vi "ResMgr-Request StatusEvent.vi"(6 "timeout in ms (5000ms)":i32=5000, 7 "WatchDogQ":refnum<queue>, 8 "Error in":errorcluster caption="Error in (no error)") -> (0 "Error out":errorcluster, 3 "Status Message":refnum<user-event>)   [LabVIEW 2017, in "Communicable State Machine.lvlib"]
uses:
  Communicable State Machine.lvlib
  Typedef/_CSM Status Change Event Data.ctl
  ResMgr-RequestDef.ctl
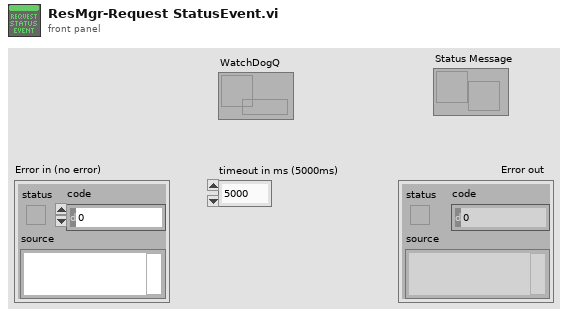
[diagram p1: front panel]
types:
  T1 = typedef "Communicable State Machine.lvlib/ResMgr-RequestDef.ctl" = cluster{"ResType":string, "RespQ":refnum<queue>, "Parameter":string, "WatchDogQ":refnum<queue>}
  T2 = typedef "Communicable State Machine.lvlib/_CSM Status Change Event Data.ctl" = cluster{"ModuleName":string, "Status":string, "Arguments":string}
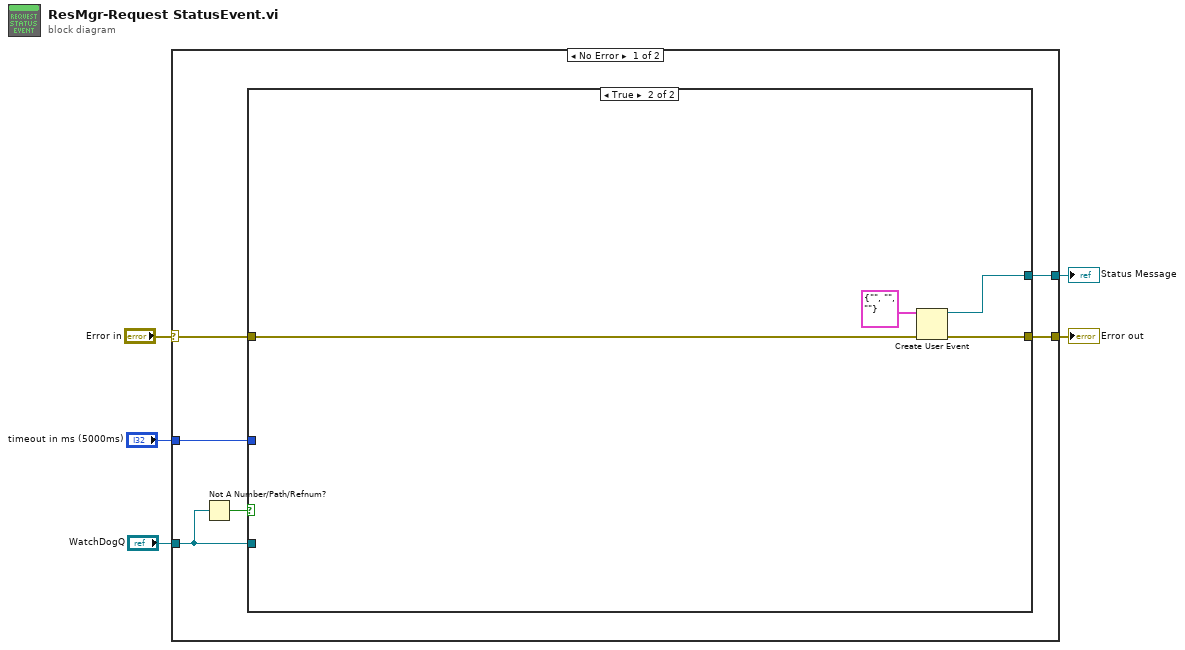
[diagram p0: block diagram]
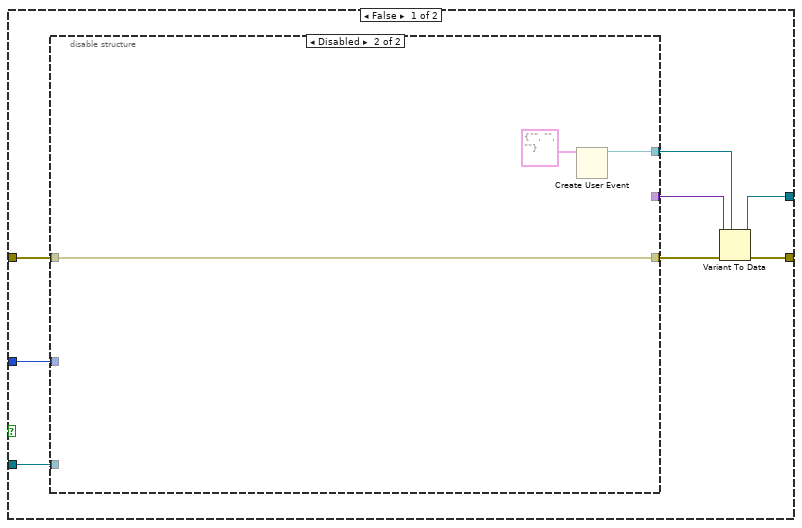
[diagram p2: hidden frame]
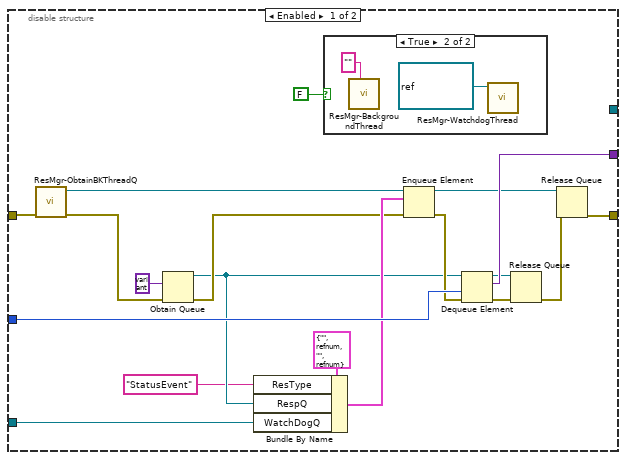
[diagram p3: hidden frame]
diagram:
  n1 = case shown="No Error" "Error in" {
    selector: "Error in" -> [w10 w48]
    tunnel: [w9 w48] -> w5
    tunnel: [w8 _] -> w1
    tunnel: "timeout in ms (5000ms)" -> [w11 _]
    tunnel: "WatchDogQ" -> [w6 _]
    frame No Error {
      n2 = Not A Number/Path/Refnum?(number/path/refnum=w6) -> (NaN/Path/Refnum?=w7:bool)
      n3 = case shown="True" w7 {
        tunnel: w11 -> [w18 _]
        tunnel: w10 -> [w17 w45]
        tunnel: w6 -> [w16 _]
        tunnel: [w15 w46] -> w9
        tunnel: [w12 w44] -> w8
        frame False {
          n4 = disable-structure shown="Disabled" {
            disable-tunnel: [w38 w43] -> w19
            disable-tunnel: w18 -> [w37 _]
            disable-tunnel: [w36 _] -> w14
            disable-tunnel: w17 -> [w20 w43]
            disable-tunnel: w16 -> [w24 _]
            disable-tunnel: [_ w41] -> w13
            frame Enabled {
              n5 = call "ResMgr-ObtainBKThreadQ.vi"("error in (no error)"=w20) -> ("error out"=w21:errorcluster, "Queue out"=w22:refnum<queue>)  [unwired: 9 in]
              n6 = Obtain Queue(element data type=variant, error in (no error)=w21) -> (queue out=w25:refnum<queue>, error out=w34:errorcluster)  [unwired: 3 in, 1 out]
              n7 = Bundle By Name(cluster=T1 {"ResType"="", "RespQ"=refnum, "Parameter"="", "WatchDogQ"=refnum} ("Cluster"), "ResType"="StatusEvent", "RespQ"=w25, "WatchDogQ"=w24) -> (w35:T1)
              n8 = case shown="True" FALSE {
                frame False {
                }
                frame True {
                  n9 = call "ResMgr-BackgroundThread.vi"("name (unnamed)"="") -> ()  [unwired: 11 in]
                  n10 = call "ResMgr-WatchdogThread.vi"("WatchDogQ"=refnum<queue> refnum) -> ()  [unwired: 11 in]
                }
              }
              n11 = Enqueue Element(queue=w22, element=w35, error in (no error)=w34) -> (queue out=w30:refnum<queue>, error out=w33:errorcluster)  [unwired: 1 in, 1 out]
              n12 = Dequeue Element(queue=w25, timeout in ms (-1)=w37, error in (no error)=w33) -> (queue out=w31:refnum<queue>, element=w36:variant, error out=w32:errorcluster)  [unwired: 1 out]
              n13 = Release Queue(queue=w31, error in (no error)=w32) -> (error out=w29:errorcluster)  [unwired: 1 in, 2 out]
              n14 = Release Queue(queue=w30, error in (no error)=w29) -> (error out=w38:errorcluster)  [unwired: 1 in, 2 out]
            }
            frame Disabled {
              n15 = Create User Event(user event datatype=T2 {"ModuleName"="", "Status"="", "Arguments"=""} ("Status Message")) -> (user event=w41:refnum<user-event>)  [unwired: 1 in, 1 out]
            }
          }
          n16 = Variant To Data(error in=w19, type=w13, Variant=w14) -> (data=w12:refnum<user-event>, error out=w15:errorcluster)
        }
        frame True {
          n17 = Create User Event(user event datatype=T2 {"ModuleName"="", "Status"="", "Arguments"=""} ("Status Message"), error in=w45) -> (user event=w44:refnum<user-event>, error out=w46:errorcluster)
        }
      }
    }
    frame Error {
    }
  }
  "Error out" <- w5
  "Status Message" <- w1
